vi "sweep_setup.vi"(11 "Sweep":T1) -> ()   [LabVIEW 2023]
uses:
  Sweep.ctl
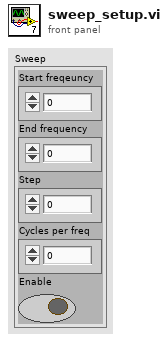
[diagram p1: front panel]
types:
  T1 = typedef "Sweep.ctl" = cluster{"Start freqeuncy":dbl, "End frequency":dbl, "Step":dbl, "Cycles per freq":dbl, "Enable":bool}
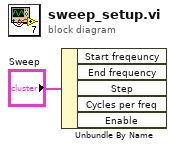
[diagram p0: block diagram]
diagram:
  n1 = Unbundle By Name("Sweep") -> ()  [unwired: 5 out]
